vi "Add Sessions to Connection Map.vi"(8 "error in":errorcluster, 10 "session info":T1[](array[typedef]), 11 "connection map in":refnum<class "Connection Map.lvclass">) -> (0 "error out":errorcluster, 3 "connection map out":refnum<class "Connection Map.lvclass">)   [LabVIEW 2020, in "MeasurementServerTests.lvlib"]
uses:
  MeasurementServerTests.lvlib
  Runtime/MeasurementLink Session Management Client/RPC Messages/ni_measurementlink_sessionmanagement_v1_SessionInformation.ctl
  Runtime/MeasurementLink Session Management Client/RPC Messages/nidevice_grpc_Session.ctl
  Runtime/MeasurementLink Session Management Client/RPC Messages/ni_measurementlink_sessionmanagement_v1_ChannelMapping.ctl
  Runtime/MeasurementLink Session Management/Connection Map/Connection Map.lvclass
  Runtime/MeasurementLink Session Management Client/MeasurementLink Session Management Client.lvlib
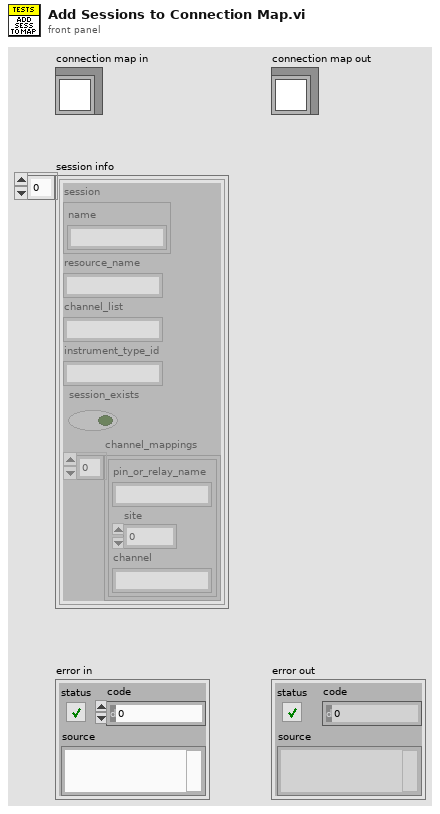
[diagram p1: front panel]
types:
  T1 = typedef "MeasurementLink Session Management Client.lvlib/ni_measurementlink_sessionmanagement_v1_SessionInformation.ctl" = cluster{"session":T2, "resource_name":string, "channel_list":string, "instrument_type_id":string, "session_exists":bool, "channel_mappings":T3[]}
  T2 = typedef "MeasurementLink Session Management Client.lvlib/nidevice_grpc_Session.ctl" = cluster{"name":string}
  T3 = typedef "MeasurementLink Session Management Client.lvlib/ni_measurementlink_sessionmanagement_v1_ChannelMapping.ctl" = cluster{"pin_or_relay_name":string, "site":i32, "channel":string}
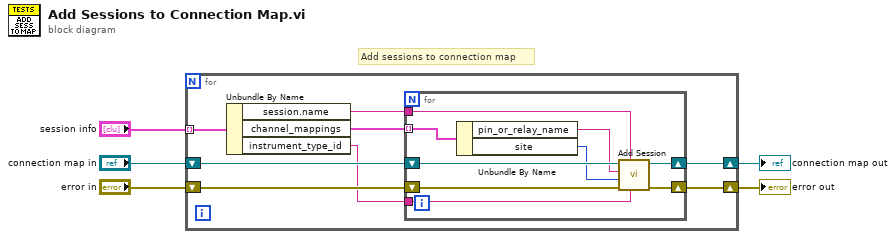
[diagram p0: block diagram]
diagram:
  # "Add sessions to connection map"
  n1 = for {
    shift-right: [w12] -> w2
    shift-left: "connection map in" -> [w13]
    shift-right: [w10] -> w4
    shift-left: "error in" -> [w11]
    tunnel: "session info" -> [w9] mode=indexing
    n2 = Unbundle By Name(w9) -> ("session.name"=w6:string, "channel_mappings"=w8:T3[], "instrument_type_id"=w7:string)
    n3 = for {
      shift-right: [w21] -> w12
      shift-left: w13 -> [w22]
      shift-right: [w19] -> w10
      shift-left: w11 -> [w20]
      tunnel: w8 -> [w18] mode=indexing
      tunnel: w7 -> [w15]
      tunnel: w6 -> [w14]
      n4 = Unbundle By Name(w18) -> ("pin_or_relay_name"=w17:string, "site"=w16:i32)
      n5 = call "Add Session.vi"("instrument type id"=w15, "session to add"=w14, "error in"=w20, "site"=w16, "pin or relay name"=w17, "connection map in"=w22) -> ("error out"=w19:errorcluster, "connection map out"=w21:refnum<class "Connection Map.lvclass">)  [unwired: 4 in]
    }
  }
  "error out" <- w4
  "connection map out" <- w2
